vi "Update Tree Item Selection.vi"(0 "TreeControl in":refnum<vi>, 5 "Measurement folder Tags":string[](array[string]), 7 "Measurement file Tags":string[](array[string]), 9 "Selected cell Tag":string, 11 "error in (no error)":errorcluster) -> (4 "TreeControl out":refnum<vi>, 15 "error out":errorcluster)   [LabVIEW 2021, in "Migrator.lvlib"]
uses:
  Migrator.lvlib
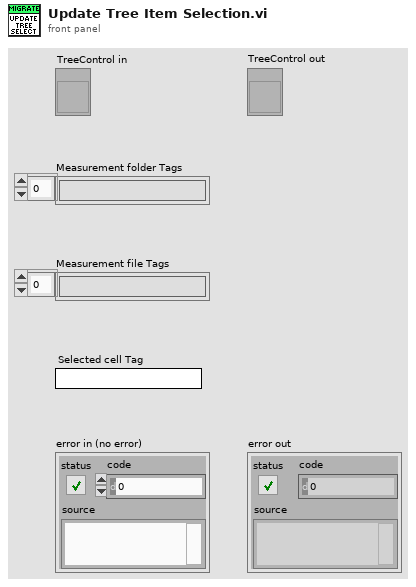
[diagram p1: front panel]
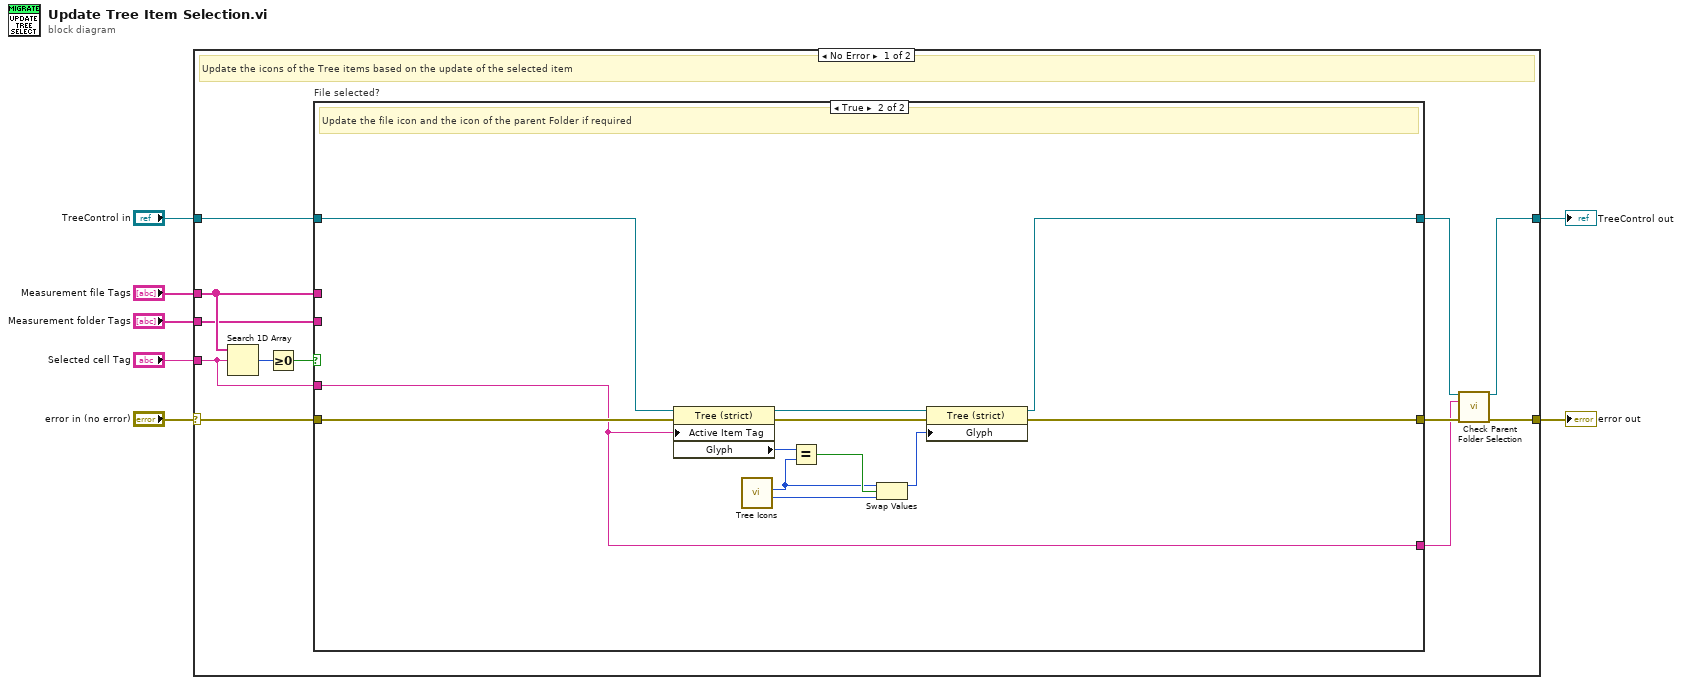
[diagram p0: block diagram]
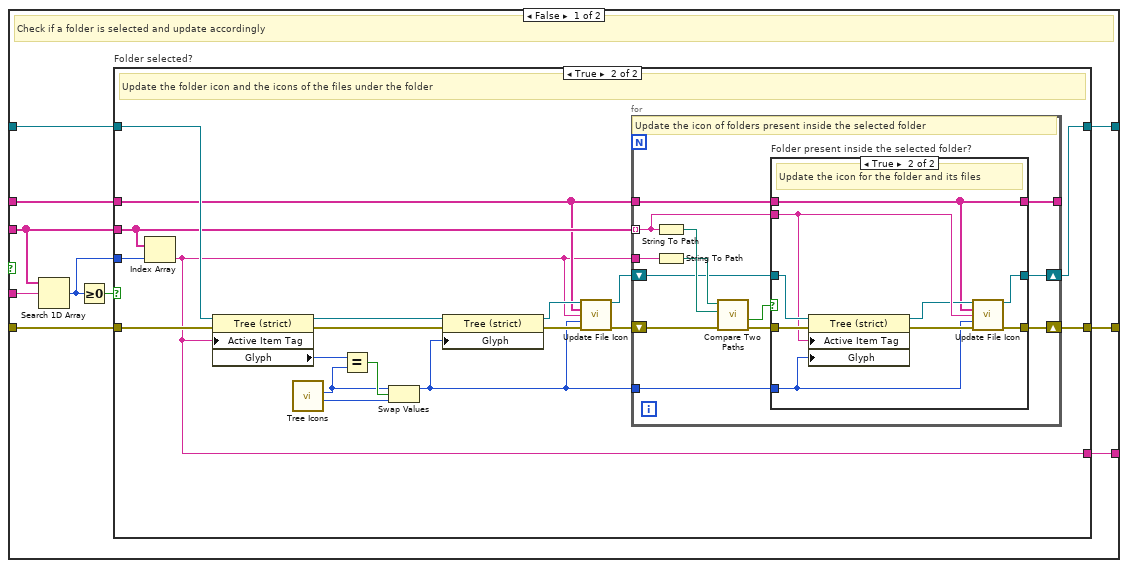
[diagram p2: hidden frame]
diagram:
  n1 = case shown="No Error" "error in (no error)" {
    selector: "error in (no error)" -> [w14 w88]
    tunnel: "Measurement file Tags" -> [w19 _]
    tunnel: "Selected cell Tag" -> [w18 _]
    tunnel: "Measurement folder Tags" -> [w17 _]
    tunnel: [w11 w88] -> w4
    tunnel: "TreeControl in" -> [w13 w89]
    tunnel: [w9 w89] -> w1
    frame No Error {
      # "Update the icons of the Tree items based on the update of the selected item"
      n2 = Search 1D Array(1D array=w19, element=w18) -> (index of element=w15:i32)  [unwired: 1 in]
      n3 = Greater Or Equal To 0?(x=w15) -> (x >= 0?=w16:bool)
      n4 = case "File selected?" shown="True" w16 {
        tunnel: w14 -> [w24 w87]
        tunnel: [w23 w78] -> w12
        tunnel: w18 -> [w29 w76]
        tunnel: w17 -> [w26 _]
        tunnel: w19 -> [w27 _]
        tunnel: w13 -> [w22 w80]
        tunnel: [w21 w77] -> w10
        tunnel: [w20 w76] -> w8
        frame False {
          # "Check if a folder is selected and update accordingly"
          n5 = Search 1D Array(1D array=w26, element=w29) -> (index of element=w25:i32)  [unwired: 1 in]
          n6 = Greater Or Equal To 0?(x=w25) -> (x >= 0?=w28:bool)
          n7 = case "Folder selected?" shown="True" w28 {
            tunnel: w27 -> [_ w36]
            tunnel: w26 -> [_ w39]
            tunnel: w25 -> [_ w50]
            tunnel: w24 -> [w31 w43]
            tunnel: [w31 w34] -> w23
            tunnel: w22 -> [w30 w42]
            tunnel: [w30 w33] -> w21
            tunnel: [_ w32] -> w20
            frame False {
              # "Pass"
            }
            frame True {
              # "Update the folder icon and the icons of the files under the folder"
              n8 = Index Array(array=w39, index=w50) -> (element=w32:string)
              n9 = property on="Property Node" class="Tree (strict)"(reference=w42, error in=w43, "Active Item Tag"=w32) -> (reference out=w44:refnum<vi>, error out=w49:errorcluster, "Glyph"=w48:i32)
              n10 = call "Tree Icons.vi"() -> ("Not Selected"=w46:i32, "Selected"=w45:i32)  [unwired: 6 in]
              n11 = Equal?(x=w48, y=w45) -> (x = y?=w47:bool)
              n12 = Swap Values(12:w45, 13:w47, 14:w46) -> (1:w38:i32)  [unwired: 1 out]
              n13 = property on="Property Node" class="Tree (strict)"(reference=w44, error in=w49, "Glyph"=w38) -> (reference out=w40:refnum<vi>, error out=w41:errorcluster)
              n14 = call "Update File Icon.vi"("TreeControl in"=w40, "Measurement file Tags"=w36, "Folder Tag"=w32, "Folder Icon"=w38, "error in (no error)"=w41) -> ("TreeControl out"=w37:refnum<vi>, "error out"=w35:errorcluster)  [unwired: 9 in]
              n15 = for {
                tunnel: w39 -> [w56] mode=indexing
                tunnel: w32 -> [w63]
                tunnel: w38 -> [w55]
                tunnel: w36 -> [w57]
                shift-right: [w54] -> w34
                shift-left: w35 -> [w53]
                shift-right: [w52] -> w33
                shift-left: w37 -> [w58]
                tunnel: [w51] -> _
                # "Update the icon of folders present inside the selected folder"
                n16 = String To Path(string=w56) -> (path=w62:path)
                n17 = String To Path(string=w63) -> (path=w61:path)
                n18 = call <vilib>:"Compare Two Paths.vi"("error in (no error)"=w53, "Path 2"=w62, "Path 1"=w61) -> ("error out"=w60:errorcluster, "Path 2 Relative to Path 1?"=w59:bool)  [unwired: 5 in, 2 out]
                n19 = case "Folder present inside the selected folder?" shown="True" w59 {
                  tunnel: w60 -> [w66 w75]
                  tunnel: w58 -> [w65 w74]
                  tunnel: w57 -> [w64 w67]
                  tunnel: w56 -> [_ w72]
                  tunnel: w55 -> [_ w71]
                  tunnel: [w66 w69] -> w54
                  tunnel: [w65 w68] -> w52
                  tunnel: [w64 w67] -> w51
                  frame False {
                    # "Pass"
                  }
                  frame True {
                    # "Update the icon for the folder and its files"
                    n20 = property on="Property Node" class="Tree (strict)"(reference=w74, error in=w75, "Active Item Tag"=w72, "Glyph"=w71) -> (reference out=w70:refnum<vi>, error out=w73:errorcluster)
                    n21 = call "Update File Icon.vi"("TreeControl in"=w70, "Measurement file Tags"=w67, "Folder Tag"=w72, "Folder Icon"=w71, "error in (no error)"=w73) -> ("TreeControl out"=w68:refnum<vi>, "error out"=w69:errorcluster)  [unwired: 9 in]
                  }
                }
              }
            }
          }
        }
        frame True {
          # "Update the file icon and the icon of the parent Folder if required"
          n22 = property on="Property Node" class="Tree (strict)"(reference=w80, error in=w87, "Active Item Tag"=w76) -> (reference out=w79:refnum<vi>, error out=w86:errorcluster, "Glyph"=w85:i32)
          n23 = call "Tree Icons.vi"() -> ("Not Selected"=w83:i32, "Selected"=w81:i32)  [unwired: 6 in]
          n24 = Equal?(x=w85, y=w81) -> (x = y?=w84:bool)
          n25 = Swap Values(12:w81, 13:w84, 14:w83) -> (1:w82:i32)  [unwired: 1 out]
          n26 = property on="Property Node" class="Tree (strict)"(reference=w79, error in=w86, "Glyph"=w82) -> (reference out=w77:refnum<vi>, error out=w78:errorcluster)
        }
      }
      n27 = call "Check Parent Folder Selection.vi"("Tree reference in"=w10, "Child Tag"=w8, "error in"=w12) -> ("Tree reference out"=w9:refnum<vi>, "error out"=w11:errorcluster)  [unwired: 11 in]
    }
    frame Error {
      # "Pass"
    }
  }
  "error out" <- w4
  "TreeControl out" <- w1
